vi "Finding Last Menaingful Position.vi"(10 "Data In":string[][](array[string])) -> (1 "Column Index":i32, 2 "Row Index":i32)   [LabVIEW 2024]
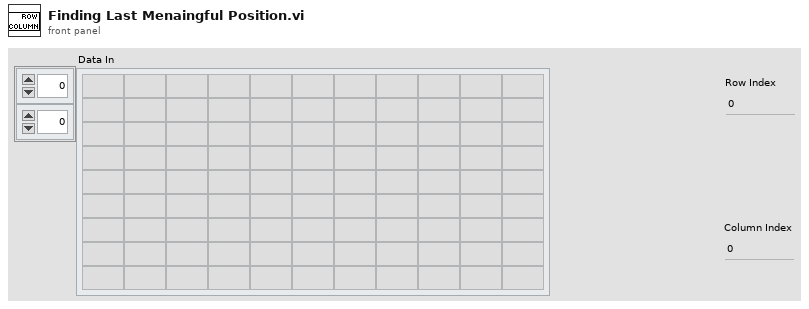
[diagram p1: front panel]
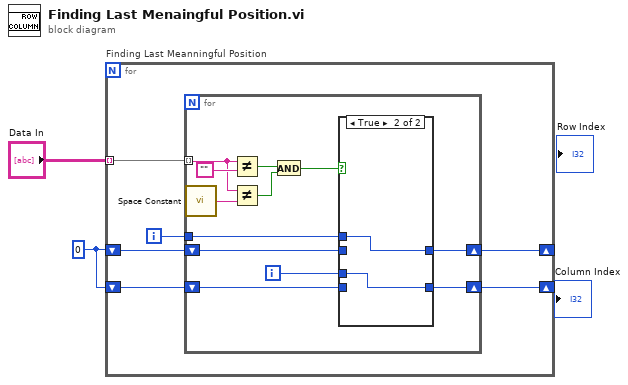
[diagram p0: block diagram]
diagram:
  w1 = 0
  n1 = for "Finding Last Meanningful Position" {
    tunnel: "Data In" -> [w8] mode=indexing
    shift-right: [w5] -> _
    shift-left: w1 -> [w7]
    shift-right: [w3] -> _
    shift-left: w1 -> [w4]
    i -> [w6]
    n2 = for {
      tunnel: w8 -> [w16] mode=indexing
      tunnel: w6 -> [w14]
      shift-right: [w13] -> w5
      shift-left: w7 -> [w12]
      shift-right: [w10] -> w3
      shift-left: w4 -> [w11]
      i -> [w9]
      n3 = call <vilib>:"Space Constant.vi"() -> ("String"=w19:string)
      n4 = Not Equal?(x=w16, y="") -> (x != y?=w18:bool)
      n5 = Not Equal?(x=w16, y=w19) -> (x != y?=w17:bool)
      n6 = And(x=w18, y=w17) -> (x .and. y?=w15:bool)
      n7 = case shown="True" w15 {
        tunnel: w14 -> [_ w24]
        tunnel: [w22 w24] -> w13
        tunnel: w12 -> [w22 _]
        tunnel: w11 -> [w21 _]
        tunnel: [w21 w23] -> w10
        tunnel: w9 -> [_ w23]
        frame False {
        }
        frame True {
        }
      }
    }
  }
